vi "Global Object Position.vi"(0 "Robot position Global":T1, 1 "Distance (m)":fxp<+/-,26,5>, 2 "Sensor Position":T2, 4 "Max Distance":dbl) -> (5 "Object position Global":cluster{"Sensor X":dbl, "Sensor Y":dbl}, 6 "Sensor position Global":cluster{"Object X":dbl, "Object Y":dbl}, 7 "In Range?":bool)   [LabVIEW 2012]
uses:
  <vilib>/Analysis/coordinate.llb/2D Cartesian Coordinate Rotation (Scalar).vi
  <vilib>/Analysis/NI_AALPro.lvlib
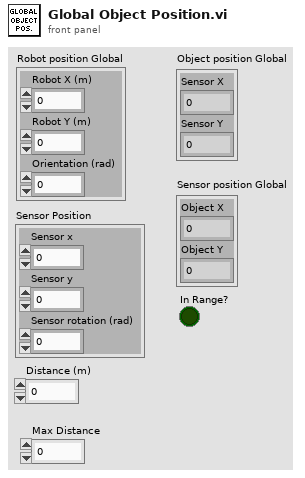
[diagram p1: front panel]
types:
  T1 = cluster{"Robot X (m)":dbl, "Robot Y (m)":dbl, "Orientation (rad)":dbl}
  T2 = cluster{"Sensor x":dbl, "Sensor y":dbl, "Sensor rotation (rad)":dbl}
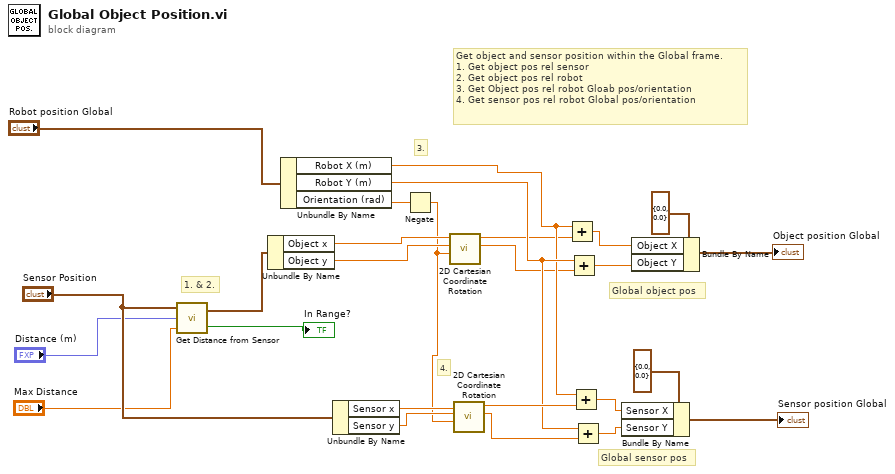
[diagram p0: block diagram]
diagram:
  # "1. & 2."
  # "Get object and sensor position within the Global frame.\n1. Get object pos rel sensor\n2. Get object pos rel robot\n3. Get Object pos rel robot Gloab pos/orientation\n4. Get sensor pos rel robot Global pos/orientation"
  # "Global object pos"
  # "Global sensor pos"
  # "4."
  # "3."
  n1 = call "Get Distance from Sensor.vi"("Max Distance"="Max Distance", "Distance (m)"="Distance (m)", "Sensor Position"="Sensor Position") -> ("In Range?"=→"In Range?":bool, "Object Position (robot)"=w6:cluster{"Object x":dbl, "Object y":dbl})
  n2 = Unbundle By Name(w6) -> ("Object x"=w9:dbl, "Object y"=w10:dbl)
  n3 = Unbundle By Name("Robot position Global") -> ("Robot X (m)"=w16:dbl, "Robot Y (m)"=w17:dbl, "Orientation (rad)"=w4:dbl)
  n4 = Unbundle By Name("Sensor Position") -> ("Sensor x"=w14:dbl, "Sensor y"=w15:dbl)
  n5 = Negate(x=w4) -> (-x=w3:dbl)
  n6 = call-poly <vilib>:"2D Cartesian Coordinate Rotation.vi"("theta"=w3, "y"=w10, "x"=w9) -> ("y out"=w13:dbl, "x out"=w12:dbl)  [unwired: 6 in, 1 out]
  n7 = call-poly <vilib>:"2D Cartesian Coordinate Rotation.vi"("theta"=w3, "y"=w15, "x"=w14) -> ("y out"=w19:dbl, "x out"=w18:dbl)  [unwired: 6 in, 1 out]
  n8 = Add(x=w16, y=w12) -> (x+y=w22:dbl)
  n9 = Add(x=w17, y=w13) -> (x+y=w23:dbl)
  n10 = Add(x=w16, y=w18) -> (x+y=w25:dbl)
  n11 = Add(x=w17, y=w19) -> (x+y=w26:dbl)
  n12 = Bundle By Name(cluster=cluster{"Sensor X":dbl, "Sensor Y":dbl} {"Sensor X"=0.0, "Sensor Y"=0.0}, "Sensor X"=w25, "Sensor Y"=w26) -> (→"Sensor position Global":cluster{"Sensor X":dbl, "Sensor Y":dbl})
  n13 = Bundle By Name(cluster=cluster{"Object X":dbl, "Object Y":dbl} {"Object X"=0.0, "Object Y"=0.0}, "Object X"=w22, "Object Y"=w23) -> (→"Object position Global":cluster{"Object X":dbl, "Object Y":dbl})
